vi "absCalcPlot_UV.vi"(4 "CRD t, t0":cluster{"crd":dbl, "tau_0 (us)":dbl}, 6 "Cell Calibration, mV/mW":dbl=600000.0, 8 "Error In":errorcluster, 9 "PD Values":cluster{dbl, dbl, dbl}, 10 "bkg values":cluster{dbl, dbl, dbl}, 11 "Mic Values":cluster{dbl, dbl, dbl}) -> (0 "Error Out":errorcluster, 1 "aae":dbl, 2 "Time Series":cluster{dbl, dbl, dbl, "b_ext (1/Mm)":dbl}, 3 "Spectrum":cluster{dbl[], "Best Power Fit":dbl[]}[](graph))   [LabVIEW 2011]
uses:
  <vilib>/Analysis/NI_AALPro.lvlib
panel:
  out "output cluster":cluster{i32[], "Best Power Fit":dbl[]}
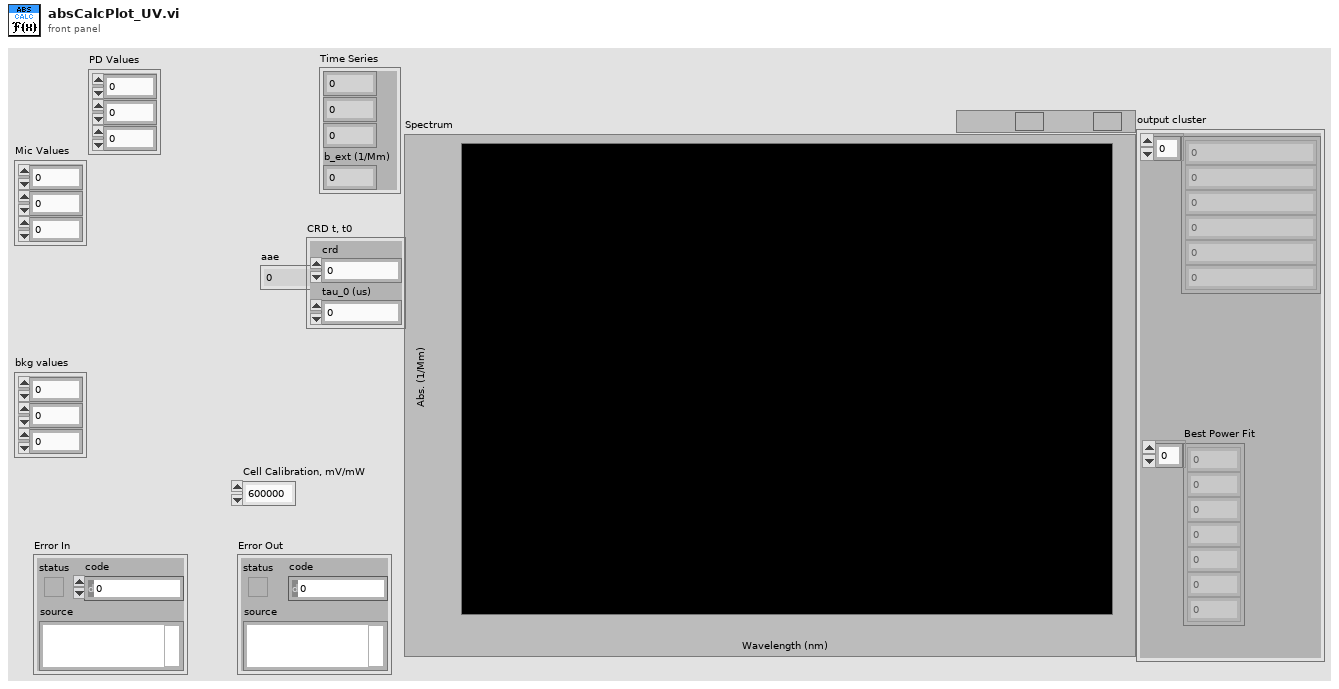
[diagram p1: front panel]
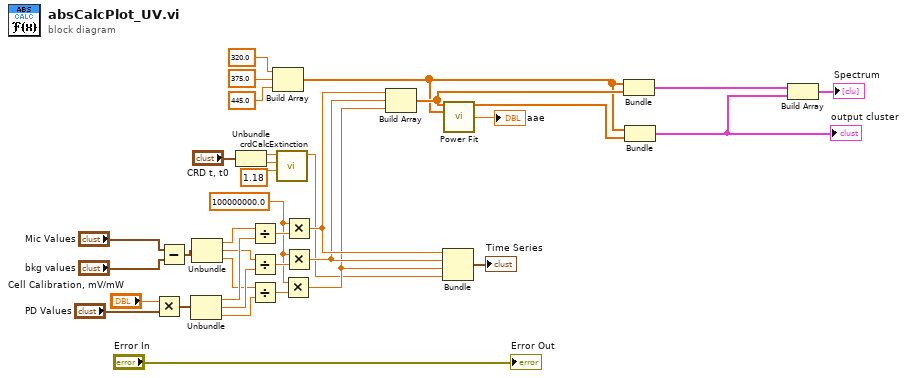
[diagram p0: block diagram]
diagram:
  w14 = 100000000.0 ("element")
  n1 = Multiply(x="Cell Calibration, mV/mW", y="PD Values") -> (x*y=w30:cluster{dbl, dbl, dbl})
  n2 = Subtract(x="Mic Values", y="bkg values") -> (x-y=w25:cluster{dbl, dbl, dbl})
  n3 = Unbundle(w30) -> (w31:dbl, w32:dbl, w33:dbl)
  n4 = Unbundle(w25) -> (w26:dbl, w27:dbl, w28:dbl)
  n5 = Unbundle("CRD t, t0") -> ("crd"=w8:dbl, "tau_0 (us)"=w7:dbl)
  n6 = Divide(x=w26, y=w31) -> (x/y=w20:dbl)
  n7 = Divide(x=w27, y=w32) -> (x/y=w19:dbl)
  n8 = Divide(x=w28, y=w33) -> (x/y=w18:dbl)
  n9 = Build Array(320.0 ("element"), 375.0 ("element"), 445.0 ("element")) -> (w16:dbl[])
  n10 = call "crdCalcExtinction.vi"("R_l"=1.18, "tau_0 (us)"=w7, "tau (us)"=w8) -> ("b_ext (1/Mm)"=w5:dbl)  [unwired: 8 in]
  n11 = Multiply(x=w14, y=w18) -> (x*y=w11:dbl)
  n12 = Multiply(x=w14, y=w20) -> (x*y=w13:dbl)
  n13 = Multiply(x=w14, y=w19) -> (x*y=w12:dbl)
  n14 = Build Array(w13, w12, w11) -> (w17:dbl[])
  n15 = Bundle(w13, w12, w11, "b_ext (1/Mm)"=w5) -> (→"Time Series":cluster{dbl, dbl, dbl, "b_ext (1/Mm)":dbl})  [unwired: 1 in]
  n16 = call <vilib>:"Power Fit.vi"("Y"=w17, "X"=w16) -> ("Best Power Fit"=w23:dbl[], "power"=→"aae":dbl)  [unwired: 8 in, 4 out]
  n17 = Bundle(w16, w17) -> (w15:cluster{dbl[], dbl[]})  [unwired: 1 in]
  n18 = Bundle(w16, "Best Power Fit"=w23) -> (w22:cluster{dbl[], "Best Power Fit":dbl[]})  [unwired: 1 in]
  "output cluster" <- w22
  n19 = Build Array(w15, w22) -> (→"Spectrum":cluster{dbl[], "Best Power Fit":dbl[]}[])
  "Error Out" <- "Error In"
